vi "Destroy.vi"(8 "error in":errorcluster, 11 "measurement service v2 in":refnum<class "Measurement Service V2.lvclass">) -> (0 "error out":errorcluster)   [LabVIEW 2020, in "Measurement Plugin Measurement Server.lvlib" / "Measurement Service V2.lvclass"]
uses:
  Measurement Service V2.lvclass
  Measurement Service V2.lvclass/Measurement Service V2.ctl
  Measurement Plugin Measurement Service Base V2/RPC Service/MeasurementService/MeasurementServiceBaseV2.lvclass
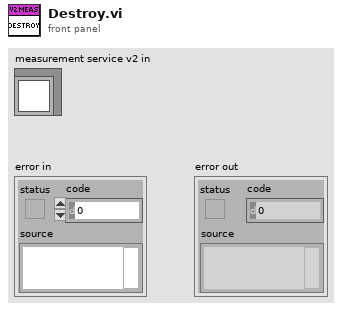
[diagram p1: front panel]
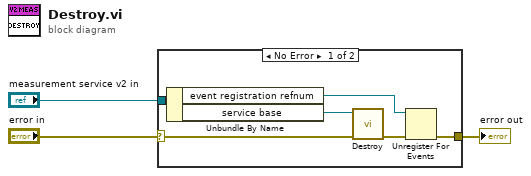
[diagram p0: block diagram]
diagram:
  n1 = case shown="No Error" "error in" {
    selector: "error in" -> [w7 w10]
    tunnel: [w5 w10] -> w2
    tunnel: "measurement service v2 in" -> [w9 _]
    frame No Error {
      n2 = Unbundle By Name(w9) -> ("event registration refnum"=w4:refnum<event-registration>, "service base"=w8:refnum<class "MeasurementServiceBaseV2.lvclass">)
      n3 = call-dynamic "Destroy.vi"("error in (no error)"=w7, "SignalGeneratorService in"=w8) -> ("error out"=w6:errorcluster)  [unwired: 8 in, 1 out]
      n4 = Unregister For Events(event registration refnum=w4, error in=w6) -> (error out=w5:errorcluster)
    }
    frame Error {
    }
  }
  "error out" <- w2
